vi "Periodic Tasks.vi"(8 "error in":errorcluster) -> ()   [LabVIEW 2017]
doc: "This VI runs in parallel to other tasks. It can contain as many user-defined periodic loops as you need. These can carry out PID or other sorts of timed response."
uses:
  <vilib>/Rock Robotics/WPI/ThirdParty/Sensors/navX/_TypeDefs/FRIC_navX_DeviceNumbersTypeDef.ctl
  <vilib>/Rock Robotics/WPI/ThirdParty/Phoenix-LabVIEW/Motor Controller/Controls/CTRE_Phoenix_MotorControl_ControlMode.ctl
  <vilib>/Rock Robotics/WPI/Utilities/WPI_GetSetVariantRefNum.vi
  <vilib>/Rock Robotics/WPI/ThirdParty/Phoenix-LabVIEW/Motor Controller/Get/CTRE_Phoenix_MotorController_GetSelectedSensorData.vi
  <vilib>/Rock Robotics/Network Tables/NT Write Number.vi
  <vilib>/Utility/file.llb/Write Delimited Spreadsheet (I64).vi
panel:
  out "Current Position Units":i32
  out "Target Position":dbl
  in  "P":dbl
  in  "D":dbl
  in  "I":dbl
  out "Zero Encoders":bool
  out "Zero Yaw":bool
  out "YRPHfH":T1
  out "Position LR (in)":dbl
  out "Position RR (in)":dbl
  out "Position LF (in)":dbl
  out "Position RF (in)":dbl
  out "Velocity LR (ft/s)":dbl format="%.2f"
  out "Position LR (Units)":i32
  out "Velocity RR (ft/s)":dbl format="%.2f"
  out "Position RR (Units)":i32
  out "Velocity LF (ft/s)":dbl format="%.2f"
  out "Position LF (Units)":i32
  out "Velocity RF (ft/s)":dbl format="%.2f"
  out "Position RF (Units)":i32
  # "ELEVATOR"
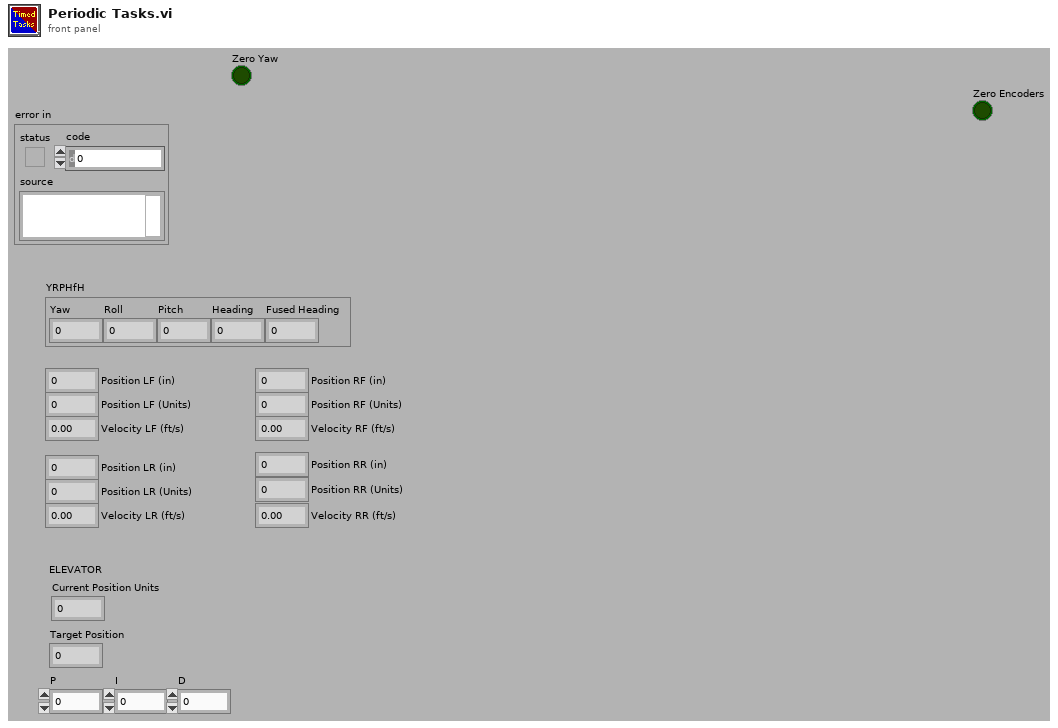
[diagram p1: front panel]
types:
  T1 = cluster{"Yaw":dbl, "Roll":dbl, "Pitch":dbl, "Heading":dbl, "Fused Heading":dbl}
  T2 = enum16{"open", "replace", "create", "open or create", "replace or create", "replace or create with confirmation"}
  T3 = typedef "WPI_JoystickDevRef.ctl" = cluster{"Device":T4}
  T4 = typedef "WPI_JoystickDeviceEnum.ctl" = enum16{"USB 0", "USB 1", "USB 2", "USB 3", "USB 4", "USB 5"}
  T5 = typedef "WPI_RobotDriveDevRef.ctl" = cluster{"DevStatus":errorcluster, "Motors[]":T6[], "Square Inputs":bool, "Max Output":dbl}
  T6 = typedef "WPI_MotorControlDeviceRef.ctl" = cluster{"DeviceStatus":errorcluster, "Type":T7, "PWM":cluster{"PWM Channel":T8, "DeadBand":T9}, "CAN":cluster{"Device Number":u8, "SetOutput VI Ref":variant, "GetOutput VI Ref":variant, "Enable VI Ref":variant, "Disable VI Ref":variant, "Data":variant}, "Invert":bool, "DIO PWM":cluster{"PWM \"Enable\" Channel":T8, "DIOChannel":T10, "PWM Rate":dbl}}
  T7 = typedef "WPI_MotorControlType.ctl" = enum16{"PWM", "CAN", "DIO PWM"}
  T8 = typedef "FPGA_DIOPWMChannel.ctl" = enum8{"PWM 0", "PWM 1", "PWM 2", "PWM 3", "PWM 4", "PWM 5", "PWM 6", "PWM 7", "PWM 8", "PWM 9", "PWM MXP 0", "PWM MXP 1", "PWM MXP 2", "PWM MXP 3", "PWM MXP 4", "PWM MXP 5", "PWM MXP 6", "PWM MXP 7", "PWM MXP 8", "PWM MXP 9", "Invalid"}
  T9 = typedef "WPI_PWMDeadband.ctl" = cluster{"Name":string, "maxPositivePwm":i32, "minPositivePwm":i32, "centerPwm":i32, "maxNegativePwm":i32, "minNegativePwm":i32, "angularRange":u16}
  T10 = typedef "FPGA_DIOChannel.ctl" = enum8{"DIO 0", "DIO 1", "DIO 2", "DIO 3", "DIO 4", "DIO 5", "DIO 6", "DIO 7", "DIO 8", "DIO 9", "DIO MXP 0", "DIO MXP 1", "DIO MXP 2", "DIO MXP 3", "DIO MXP 4", "DIO MXP 5", "DIO MXP 6", "DIO MXP 7", "DIO MXP 8", "DIO MXP 9", "DIO MXP 10", "DIO MXP 11", "DIO MXP 12", "DIO MXP 13", "DIO MXP 14", "DIO MXP 15", "SPI Port CS1", "SPI Port CS2", "SPI Port CS3", "SPI Port MISO", "SPI Port MOSI", "Invalid"}
  T11 = cluster{"JoystickDevRef":T3, "RobotDriveDevRef":T5}
  T12 = cluster{"POVs[0]":i16, "POVs[1]":i16, "POVs[2]":i16, "POVs[3]":i16, "POVs[4]":i16, "POVs[5]":i16, "POVs[6]":i16, "POVs[7]":i16, "POVs[8]":i16}
  T13 = cluster{"Buttons[0]":bool, "Buttons[1]":bool, "Buttons[2]":bool, "Buttons[3]":bool, "Buttons[4]":bool, "Buttons[5]":bool, "Buttons[6]":bool, "Buttons[7]":bool, "Buttons[8]":bool}
  T14 = typedef "CTRE_Phoenix_MotorControl_ControlMode.ctl" = u16
  T15 = typedef "FRIC_navX_DeviceNumbersTypeDef.ctl" = enum16{"Dev0", "Dev1", "Dev2", "Dev3"}
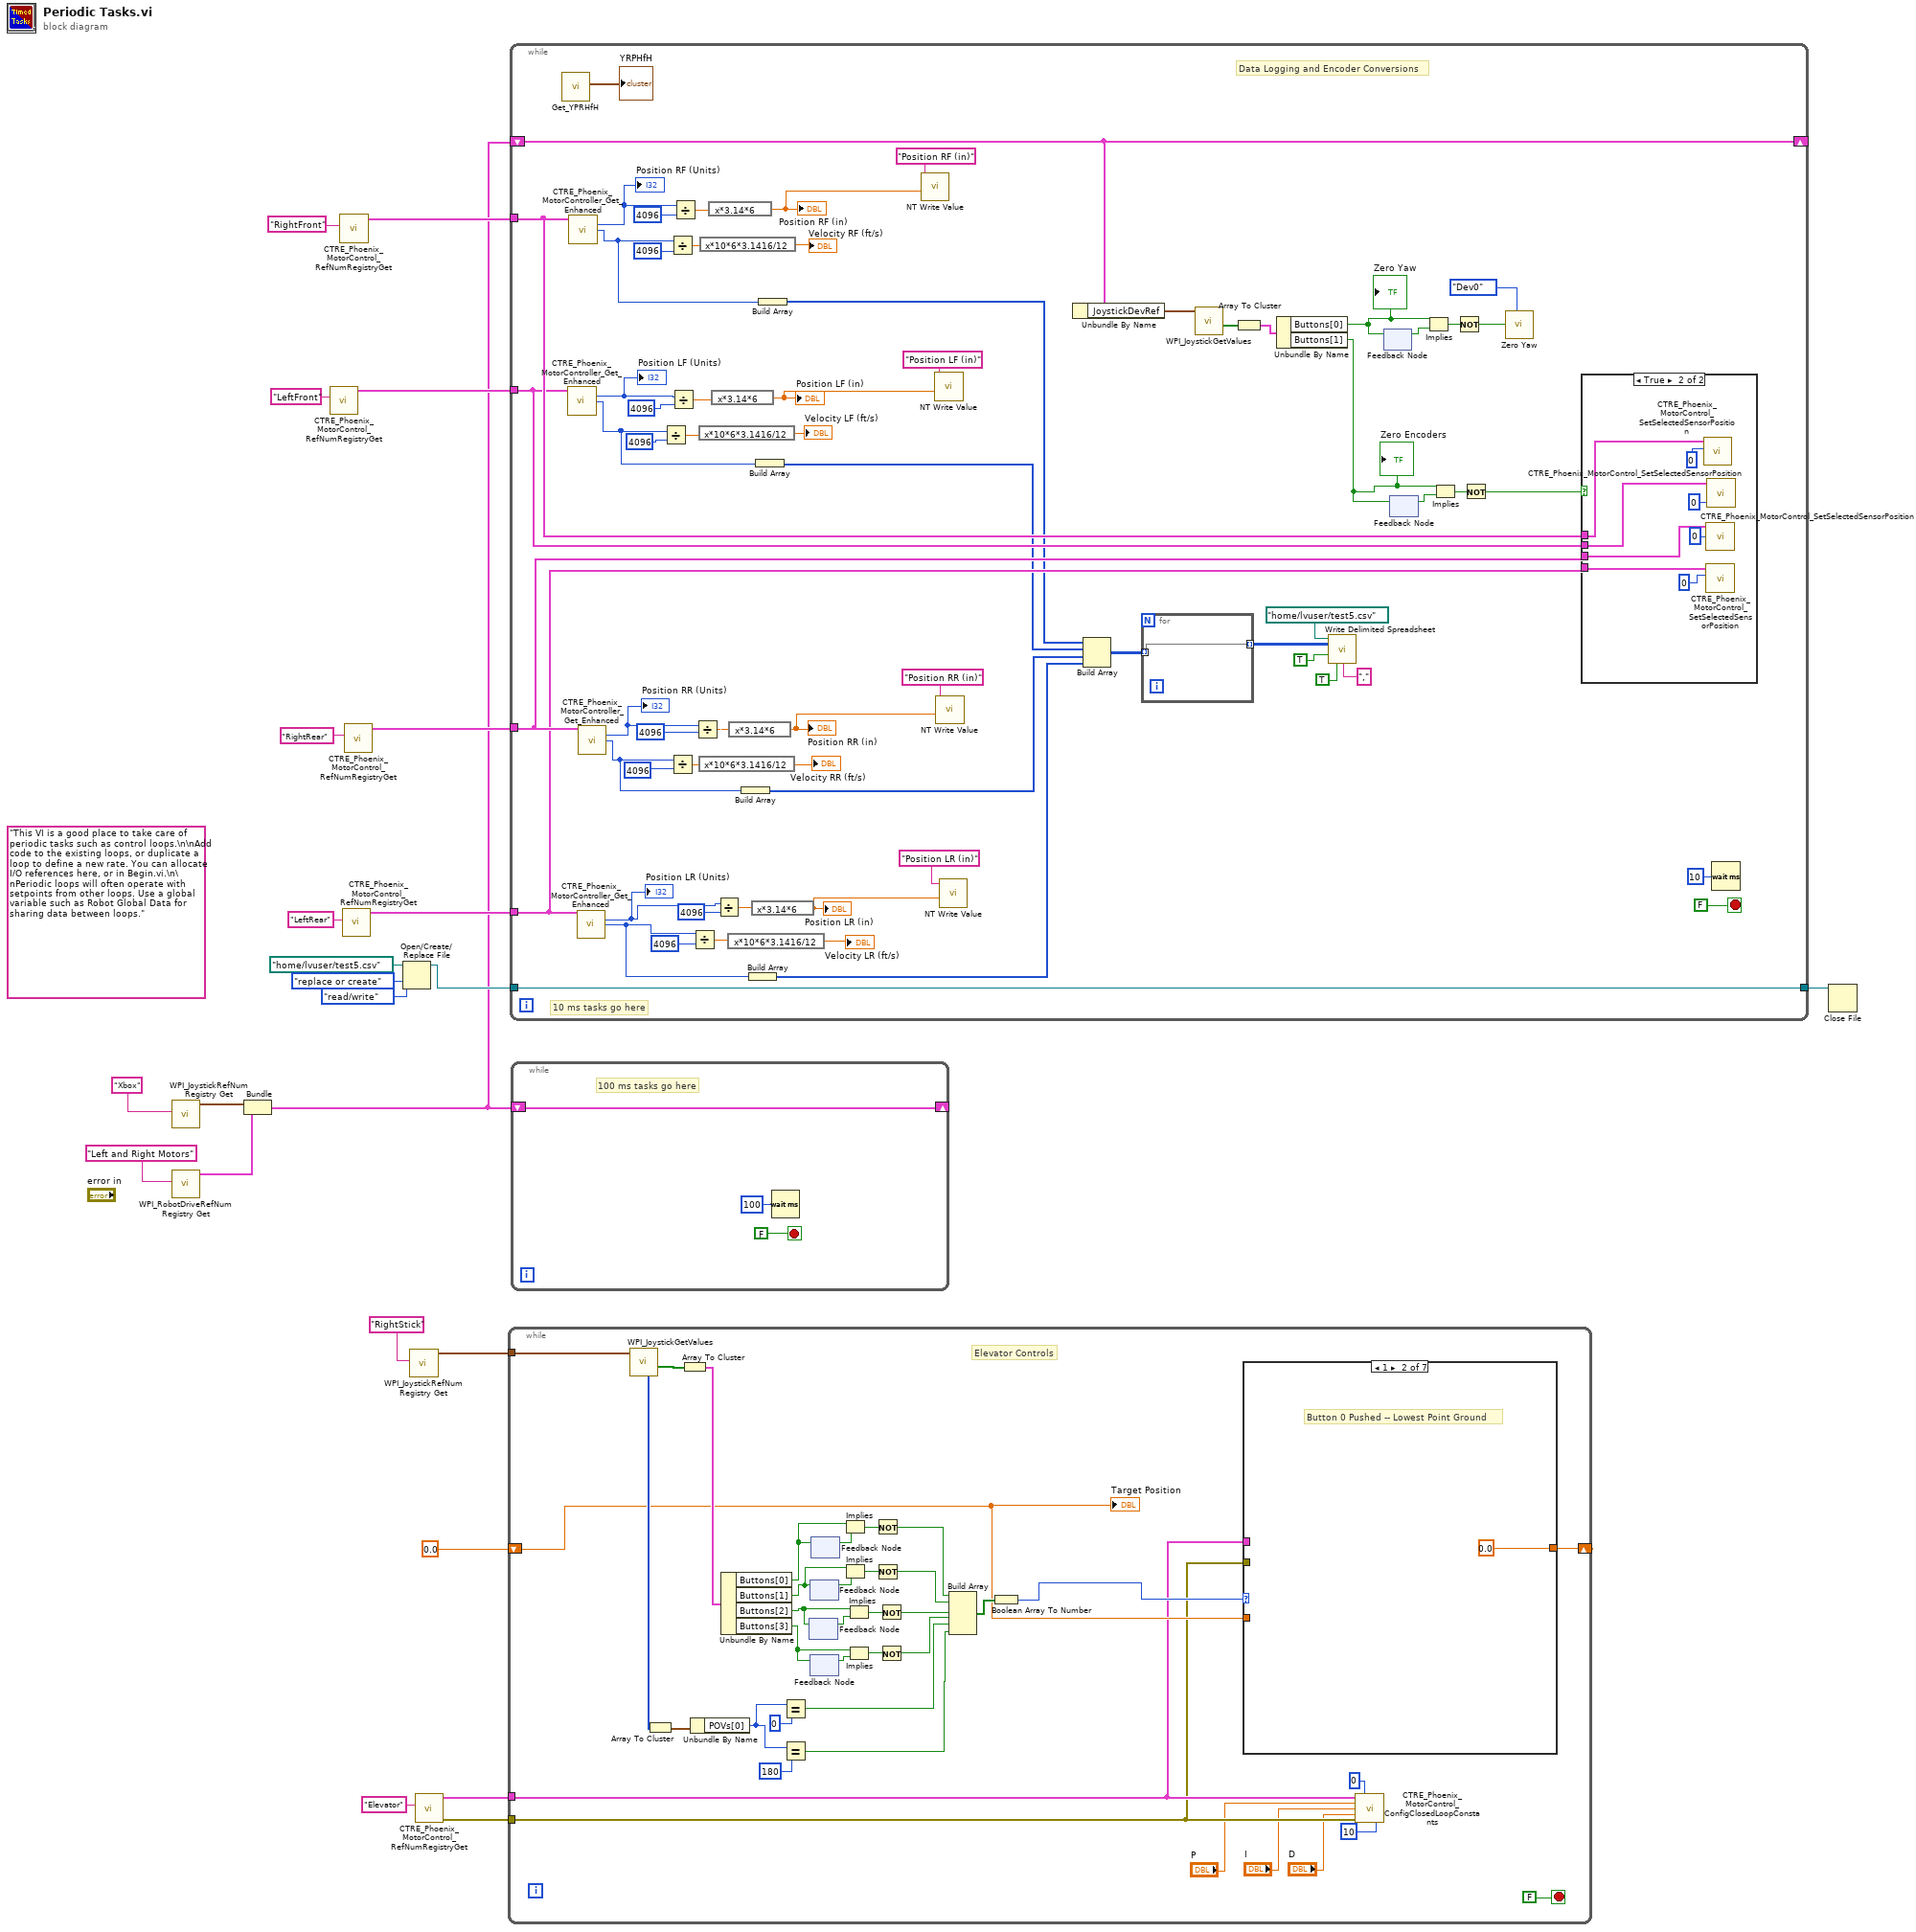
[diagram p0: block diagram]
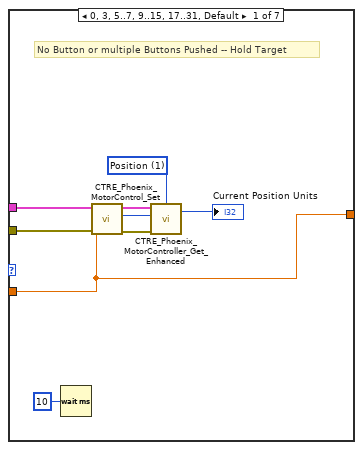
[diagram p2: hidden frame]
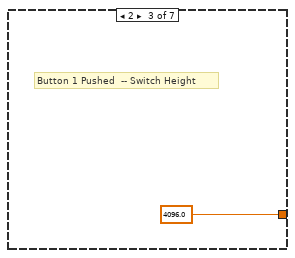
[diagram p3: hidden frame]
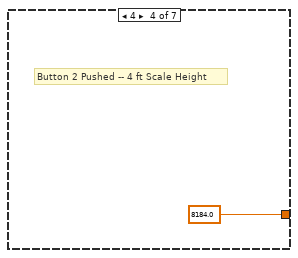
[diagram p4: hidden frame]
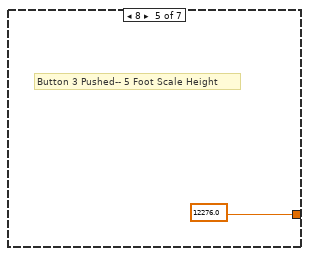
[diagram p5: hidden frame]
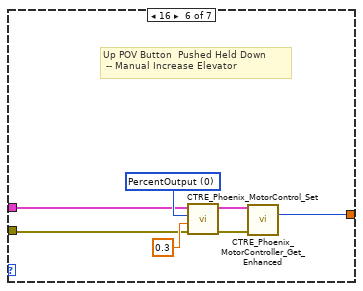
[diagram p6: hidden frame]
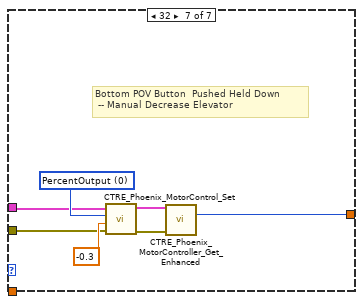
[diagram p7: hidden frame]
diagram:
  (unwired) "This VI is a good place to take care of periodic tasks such as control loops.\n\nAdd code to the existing loops, or duplicate a loop to define a new rate. You can allocate I/O references here, or in Begin.vi.\n\nPeriodic loops will often operate with setpoints from other loops. Use a global variable such as Robot Global Data for sharing data between loops."
  n1 = call <vilib>:"WPI_JoystickRefNum Registry Get.vi"("refnum name"="Xbox") -> ("JoystickDevRef"=w22:T3)  [unwired: 1 in, 9 out]
  n2 = call <vilib>:"WPI_RobotDriveRefNum Registry Get.vi"("refnum name"="Left and Right Motors") -> ("RobotDriveDevRef"=w21:T5)  [unwired: 1 in, 9 out]
  n3 = Bundle("JoystickDevRef"=w22, "RobotDriveDevRef"=w21) -> (w3:T11)  [unwired: 1 out]
  n4 = call <vilib>:"CTRE_Phoenix_MotorControl_RefNumRegistryGet.vi"("refnum name"="LeftFront") -> ("PhoenixMotorControlDevRef"=w15:T6)  [unwired: 9 in, 1 out]
  n5 = call <vilib>:"CTRE_Phoenix_MotorControl_RefNumRegistryGet.vi"("refnum name"="RightFront") -> ("PhoenixMotorControlDevRef"=w16:T6)  [unwired: 9 in, 1 out]
  n6 = call <vilib>:"CTRE_Phoenix_MotorControl_RefNumRegistryGet.vi"("refnum name"="LeftRear") -> ("PhoenixMotorControlDevRef"=w13:T6)  [unwired: 9 in, 1 out]
  n7 = call <vilib>:"CTRE_Phoenix_MotorControl_RefNumRegistryGet.vi"("refnum name"="RightRear") -> ("PhoenixMotorControlDevRef"=w14:T6)  [unwired: 9 in, 1 out]
  n8 = Open/Create/Replace File(file path (use dialog)=path "/home/lvuser/test5.csv", operation (0:open)=T2."replace or create", access (0:read/write)=enum16{"read/write", "read-only", "write-only"}."read/write") -> (refnum out=w9:refnum<file>)  [unwired: 3 in, 2 out]
  n9 = call <vilib>:"WPI_JoystickRefNum Registry Get.vi"("refnum name"="RightStick") -> ("JoystickDevRef"=w1:T3)  [unwired: 1 in, 9 out]
  n10 = call <vilib>:"CTRE_Phoenix_MotorControl_RefNumRegistryGet.vi"("refnum name"="Elevator") -> ("error out"=w5:errorcluster, "PhoenixMotorControlDevRef"=w4:T6)  [unwired: 9 in]
  n11 = while {
    shift-right: [w58] -> _
    shift-left: 0.0 -> [w52]
    tunnel: w5 -> [w50]
    tunnel: w4 -> [w51]
    tunnel: w1 -> [w25]
    stop <- FALSE stop-if-true
    # "Elevator Controls"
    n12 = call <vilib>:"WPI_JoystickGetValues.vi"("JoystickDevRef"=w25) -> ("Buttons"=w62:bool[], "POVs"=w57:i16[])  [unwired: 6 in, 3 out]
    n13 = Array To Cluster(array=w57) -> (cluster=w56:T12)
    n14 = Array To Cluster(array=w62) -> (cluster=w61:T13)
    n15 = Unbundle By Name(w56) -> ("POVs[0]"=w54:i16)
    n16 = Unbundle By Name(w61) -> ("Buttons[0]"=w41:bool, "Buttons[1]"=w36:bool, "Buttons[2]"=w31:bool, "Buttons[3]"=w27:bool)
    n17 = Equal?(x=w54, y=i16 0) -> (x = y?=w43:bool)
    n18 = Equal?(x=w54, y=i16 180) -> (x = y?=w34:bool)
    n19 = feedback #1() -> (w33:bool)  [unwired: 1 in]
    n20 = feedback-in #1(w31) -> ()
    n21 = feedback #2() -> (w38:bool)  [unwired: 1 in]
    n22 = feedback-in #2(w36) -> ()
    n23 = feedback #3() -> (w29:bool)  [unwired: 1 in]
    n24 = feedback-in #3(w27) -> ()
    n25 = feedback #4() -> (w40:bool)  [unwired: 1 in]
    n26 = feedback-in #4(w41) -> ()
    n27 = Implies(1:w40, 2:w41) -> (0:w42:bool)
    n28 = Implies(1:w38, 2:w36) -> (0:w37:bool)
    n29 = Implies(1:w33, 2:w31) -> (0:w32:bool)
    n30 = Implies(1:w29, 2:w27) -> (0:w28:bool)
    n31 = Not(x=w42) -> (.not. x?=w39:bool)
    n32 = Not(x=w37) -> (.not. x?=w35:bool)
    n33 = Not(x=w32) -> (.not. x?=w30:bool)
    n34 = Not(x=w28) -> (.not. x?=w26:bool)
    n35 = Build Array(w39, w35, w30, w26, w43, w34) -> (w60:bool[])
    n36 = Boolean Array To Number(Boolean array=w60) -> (number=w59:u32)
    n37 = case shown="1" w59 {
      tunnel: w52 -> [w63 _ _ _ _ _ _]
      tunnel: [w63 0.0 4096.0 8184.0 12276.0 w77 w84] -> w58
      tunnel: w51 -> [w68 _ _ _ _ w76 w83]
      tunnel: w50 -> [w69 _ _ _ _ w75 w82]
      frame 0, 3, 5..7, 9..15, 17..31, Default {
        w70 = T14 1 items=["PercentOutput"=0, "Position"=1, "Velocity"=2, "Current"=3, "Follower"=5, "MotionProfile"=6, "MotionMagic"=7, "MotionMagicArc"=8, "MotionProfileArc"=10, "Disabled"=15] ("Control Mode")
        # "No Button or multiple Buttons Pushed -- Hold Target"
        n38 = Wait (ms)(milliseconds to wait=u32 10) -> ()  [unwired: 1 out]
        n39 = call <vilib>:"CTRE_Phoenix_MotorControl_Set.vi"("error in (no error)"=w69, "Output"=w63, "Control Mode"=w70, "PhoenixMotorControlDevRef"=w68) -> ("error out"=w65:errorcluster, "PhoenixMotorControlDevRef"=w66:T6)  [unwired: 6 in]
        n40 = call-poly <vilib>:"CTRE_Phoenix_MotorController_Get_Enhanced.vi"("PhoenixMotorControlDevRef"=w66, "error in"=w65) -> ("Position (Raw Sensor Units)"=→"Current Position Units":i32)  [unwired: 10 in, 3 out]
      }
      frame 1 {
        # "Button 0 Pushed -- Lowest Point Ground"
      }
      frame 2 {
        # "Button 1 Pushed  -- Switch Height"
      }
      frame 4 {
        # "Button 2 Pushed -- 4 ft Scale Height"
      }
      frame 8 {
        # "Button 3 Pushed-- 5 Foot Scale Height"
      }
      frame 16 {
        w81 = T14 0 items=["PercentOutput"=0, "Position"=1, "Velocity"=2, "Current"=3, "Follower"=5, "MotionProfile"=6, "MotionMagic"=7, "MotionMagicArc"=8, "MotionProfileArc"=10, "Disabled"=15] ("Control Mode")
        # "Up POV Button  Pushed Held Down\n -- Manual Increase Elevator"
        n41 = call <vilib>:"CTRE_Phoenix_MotorControl_Set.vi"("error in (no error)"=w75, "Output"=0.3, "Control Mode"=w81, "PhoenixMotorControlDevRef"=w76) -> ("error out"=w79:errorcluster, "PhoenixMotorControlDevRef"=w80:T6)  [unwired: 6 in]
        n42 = call-poly <vilib>:"CTRE_Phoenix_MotorController_Get_Enhanced.vi"("PhoenixMotorControlDevRef"=w80, "error in"=w79) -> ("Position (Raw Sensor Units)"=w77:i32)  [unwired: 10 in, 3 out]
      }
      frame 32 {
        w88 = T14 0 items=["PercentOutput"=0, "Position"=1, "Velocity"=2, "Current"=3, "Follower"=5, "MotionProfile"=6, "MotionMagic"=7, "MotionMagicArc"=8, "MotionProfileArc"=10, "Disabled"=15] ("Control Mode")
        # "Bottom POV Button  Pushed Held Down\n -- Manual Decrease Elevator"
        n43 = call <vilib>:"CTRE_Phoenix_MotorControl_Set.vi"("error in (no error)"=w82, "Output"=-0.3, "Control Mode"=w88, "PhoenixMotorControlDevRef"=w83) -> ("error out"=w86:errorcluster, "PhoenixMotorControlDevRef"=w87:T6)  [unwired: 6 in]
        n44 = call-poly <vilib>:"CTRE_Phoenix_MotorController_Get_Enhanced.vi"("PhoenixMotorControlDevRef"=w87, "error in"=w86) -> ("Position (Raw Sensor Units)"=w84:i32)  [unwired: 10 in, 3 out]
      }
    }
    n45 = call <vilib>:"CTRE_Phoenix_MotorControl_ConfigClosedLoopConstants.vi"("PhoenixMotorControlDevRef"=w51, "slotIdx"=0, "P"="P", "I"="I", "D"="D", "error in (no error)"=w50, "timeoutMs"=10) -> ()  [unwired: 7 in, 2 out]
    "Target Position" <- w52
  }
  n46 = while {
    shift-right: [w120] -> _
    shift-left: w3 -> [w120]
    tunnel: w16 -> [w108]
    tunnel: w15 -> [w107]
    tunnel: w14 -> [w106]
    tunnel: w13 -> [w105]
    tunnel: w9 -> [w90]
    tunnel: [w90] -> w8
    stop <- FALSE stop-if-true
    # "Data Logging and Encoder Conversions"
    # "10 ms tasks go here"
    n47 = call <vilib>:"Get_YPRHfH.vi"() -> ("YRPHfH"=→"YRPHfH":T1)  [unwired: 11 in]
    n48 = call-poly <vilib>:"CTRE_Phoenix_MotorController_Get_Enhanced.vi"("PhoenixMotorControlDevRef"=w107) -> ("Position (Raw Sensor Units)"=w148:i32, "Velocity (Raw Sensor Units per 100 ms)"=w96:i32)  [unwired: 11 in, 2 out]
    "Position LF (Units)" <- w148
    n49 = call-poly <vilib>:"CTRE_Phoenix_MotorController_Get_Enhanced.vi"("PhoenixMotorControlDevRef"=w108) -> ("Position (Raw Sensor Units)"=w153:i32, "Velocity (Raw Sensor Units per 100 ms)"=w95:i32)  [unwired: 11 in, 2 out]
    "Position RF (Units)" <- w153
    n50 = call-poly <vilib>:"CTRE_Phoenix_MotorController_Get_Enhanced.vi"("PhoenixMotorControlDevRef"=w105) -> ("Position (Raw Sensor Units)"=w142:i32, "Velocity (Raw Sensor Units per 100 ms)"=w99:i32)  [unwired: 11 in, 2 out]
    "Position LR (Units)" <- w142
    n51 = call-poly <vilib>:"CTRE_Phoenix_MotorController_Get_Enhanced.vi"("PhoenixMotorControlDevRef"=w106) -> ("Position (Raw Sensor Units)"=w138:i32, "Velocity (Raw Sensor Units per 100 ms)"=w97:i32)  [unwired: 11 in, 2 out]
    "Position RR (Units)" <- w138
    n52 = Divide(x=w96, y=4096) -> (x/y=w126:dbl)
    n53 = Divide(x=w95, y=4096) -> (x/y=w124:dbl)
    n54 = Divide(x=w97, y=4096) -> (x/y=w128:dbl)
    n55 = Divide(x=w148, y=4096) -> (x/y=w135:dbl)
    n56 = Divide(x=w153, y=4096) -> (x/y=w133:dbl)
    n57 = Divide(x=w99, y=4096) -> (x/y=w130:dbl)
    n58 = Divide(x=w138, y=4096) -> (x/y=w136:dbl)
    n59 = expression code="x*10*6*3.1416/12"(w126) -> (→"Velocity LF (ft/s)":dbl)
    n60 = expression code="x*10*6*3.1416/12"(w128) -> (→"Velocity RR (ft/s)":dbl)
    n61 = expression code="x*10*6*3.1416/12"(w124) -> (→"Velocity RF (ft/s)":dbl)
    n62 = expression code="x*3.14*6"(w133) -> (w132:dbl)
    "Position RF (in)" <- w132
    n63 = expression code="x*3.14*6"(w135) -> (w134:dbl)
    "Position LF (in)" <- w134
    n64 = Divide(x=w142, y=4096) -> (x/y=w140:dbl)
    n65 = expression code="x*10*6*3.1416/12"(w130) -> (→"Velocity LR (ft/s)":dbl)
    n66 = expression code="x*3.14*6"(w136) -> (w139:dbl)
    "Position RR (in)" <- w139
    n67 = Build Array(w97) -> (w92:i32[])
    n68 = Build Array(w99) -> (w98:i32[])
    n69 = expression code="x*3.14*6"(w140) -> (w129:dbl)
    "Position LR (in)" <- w129
    n70 = Build Array(w96) -> (w93:i32[])
    n71 = Build Array(w95) -> (w94:i32[])
    n72 = call-poly <vilib>:"NT Write Value.vi"("Numeric"=w132, "Name"="Position RF (in)") -> ()  [unwired: 9 in, 1 out]
    n73 = call-poly <vilib>:"NT Write Value.vi"("Numeric"=w134, "Name"="Position LF (in)") -> ()  [unwired: 9 in, 1 out]
    n74 = call-poly <vilib>:"NT Write Value.vi"("Numeric"=w139, "Name"="Position RR (in)") -> ()  [unwired: 9 in, 1 out]
    n75 = call-poly <vilib>:"NT Write Value.vi"("Numeric"=w129, "Name"="Position LR (in)") -> ()  [unwired: 9 in, 1 out]
    n76 = Unbundle By Name(w120) -> ("JoystickDevRef"=w119:T3)
    n77 = Build Array(w94, w93, w92, w98) -> (w100:i32[][])
    n78 = for {
      tunnel: [w156] -> w91 mode=indexing
      tunnel: w100 -> [w156] mode=indexing
    }
    n79 = call <vilib>:"WPI_JoystickGetValues.vi"("JoystickDevRef"=w119) -> ("Buttons"=w118:bool[])  [unwired: 6 in, 4 out]
    n80 = Array To Cluster(array=w118) -> (cluster=w117:T13)
    n81 = Unbundle By Name(w117) -> ("Buttons[0]"=w116:bool, "Buttons[1]"=w110:bool)
    "Zero Yaw" <- w116
    "Zero Encoders" <- w110
    n82 = call-poly <vilib>:"Write Delimited Spreadsheet.vi"("file path (dialog if empty)"=path "/home/lvuser/test5.csv", "2D data"=w91, "append to file? (new file:F)"=TRUE, "transpose? (no:F)"=TRUE, "delimiter (\\t)"="," ("delimiter (\\t)")) -> ()  [unwired: 9 in, 2 out]
    n83 = feedback #5() -> (w121:bool)  [unwired: 1 in]
    n84 = feedback-in #5(w116) -> ()
    n85 = feedback #6() -> (w111:bool)  [unwired: 1 in]
    n86 = feedback-in #6(w110) -> ()
    n87 = Implies(1:w121, 2:w116) -> (0:w122:bool)
    n88 = Implies(1:w111, 2:w110) -> (0:w112:bool)
    n89 = Not(x=w122) -> (.not. x?=w115:bool)
    n90 = Not(x=w112) -> (.not. x?=w109:bool)
    n91 = call <vilib>:"Zero Yaw.vi"("Device Number"=FRIC_navX_DeviceNumbersTypeDef."Dev0", "Zero"=w115) -> ()  [unwired: 10 in]
    n92 = case shown="True" w109 {
      tunnel: w108 -> [_ w160]
      tunnel: w107 -> [_ w159]
      tunnel: w106 -> [_ w158]
      tunnel: w105 -> [_ w157]
      frame False {
      }
      frame True {
        n93 = call <vilib>:"CTRE_Phoenix_MotorControl_SetSelectedSensorPosition.vi"("New Sensor Position"=0, "PhoenixMotorControlDevRef"=w160) -> ()  [unwired: 8 in, 2 out]
        n94 = call <vilib>:"CTRE_Phoenix_MotorControl_SetSelectedSensorPosition.vi"("New Sensor Position"=0, "PhoenixMotorControlDevRef"=w158) -> ()  [unwired: 8 in, 2 out]
        n95 = call <vilib>:"CTRE_Phoenix_MotorControl_SetSelectedSensorPosition.vi"("New Sensor Position"=0, "PhoenixMotorControlDevRef"=w157) -> ()  [unwired: 8 in, 2 out]
        n96 = call <vilib>:"CTRE_Phoenix_MotorControl_SetSelectedSensorPosition.vi"("New Sensor Position"=0, "PhoenixMotorControlDevRef"=w159) -> ()  [unwired: 8 in, 2 out]
      }
    }
    n97 = Wait (ms)(milliseconds to wait=u32 10) -> ()  [unwired: 1 out]
  }
  n98 = while {
    shift-right: [w165] -> _
    shift-left: w3 -> [w165]
    stop <- FALSE stop-if-true
    # "100 ms tasks go here"
    n99 = Wait (ms)(milliseconds to wait=u32 100) -> ()  [unwired: 1 out]
  }
  n100 = Close File(refnum=w8) -> ()  [unwired: 1 in, 2 out]
